vi "Read Flattened Data.vi"(9 "Count":i32, 11 "Stream in":refnum<class "Stream.lvclass">) -> (0 "error out":errorcluster, 2 "Data":string, 3 "Stream out":refnum<class "Stream.lvclass">)   [LabVIEW 2020, in "Stream.lvlib" / "Stream.lvclass"]
uses:
  Stream.lvclass
  Data Direction.ctl
  Stream.lvlib
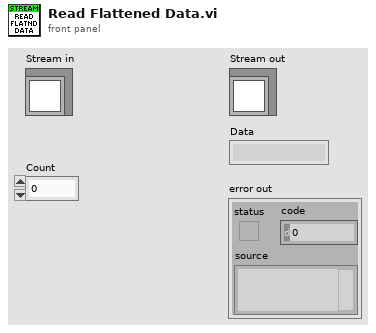
[diagram p1: front panel]
types:
  T1 = typedef "Stream.lvlib/Data Direction.ctl" = enum16{"Incoming", "Outgoing"}
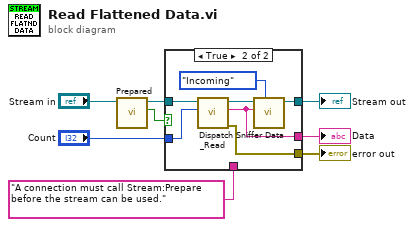
[diagram p0: block diagram]
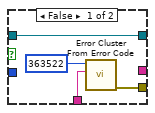
[diagram p2: hidden frame]
diagram:
  n1 = call "Prepared.vi"("Stream in"="Stream in") -> ("Prepared"=w6:bool, "Stream out"=w7:refnum<class "Stream.lvclass">)  [unwired: 8 in, 1 out]
  n2 = case shown="True" w6 {
    tunnel: "Count" -> [_ w19]
    tunnel: [w11 w18] -> w2
    tunnel: [_ w13] -> w1
    tunnel: [w12 w15] -> w5
    tunnel: w7 -> [w12 w14]
    tunnel: "A connection must call Stream:Prepare before the stream can be used." ("error message (\"\")") -> [w9 _]
    frame False {
      n3 = call <vilib>:"Error Cluster From Error Code.vi"("error message (\"\")"=w9, "error code (0)"=363522) -> ("error out"=w11:errorcluster)  [unwired: 7 in]
    }
    frame True {
      n4 = call-dynamic "_Read.vi"("Count"=w19, "Stream in"=w14) -> ("error out"=w18:errorcluster, "Data"=w13:string, "Stream out"=w17:refnum<class "Stream.lvclass">)  [unwired: 7 in]
      n5 = call "Dispatch Sniffer Data.vi"("Data Direction"=Data_Direction."Incoming", "Data"=w13, "Stream in"=w17) -> ("Stream out"=w15:refnum<class "Stream.lvclass">)  [unwired: 7 in, 1 out]
    }
  }
  "error out" <- w2
  "Stream out" <- w5
  "Data" <- w1
